vi "Write GObjects.vi"(5 "GObjects":variant, 9 "VI Interpreter in":refnum<class "VI Interpreter.lvclass">) -> (3 "VI Interpreter out":refnum<class "VI Interpreter.lvclass">)   [LabVIEW 2014, in "Raspberry Pi Compatible Compiler for LabVIEW.lvlib" / "VI Interpreter.lvclass"]
uses:
  VI Interpreter.lvclass
  VI Interpreter.lvclass/VI Interpreter.ctl
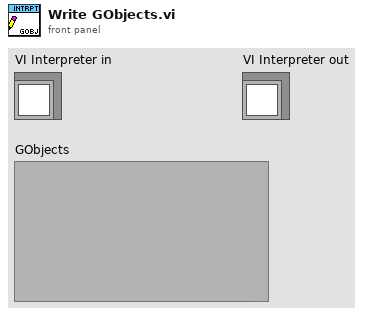
[diagram p1: front panel]
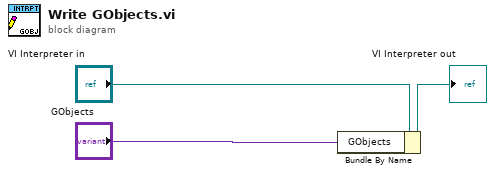
[diagram p0: block diagram]
diagram:
  n1 = Bundle By Name(cluster="VI Interpreter in", "GObjects"="GObjects") -> (→"VI Interpreter out":refnum<class "VI Interpreter.lvclass">)
